vi "GetSourceOutput.vi"(7 "SMU":T1, 8 "Error In":errorcluster, 11 "Kiethley 2602 In":refnum<visa-resource-name>) -> (0 "Error Out":errorcluster, 2 "Enabled?":bool, 3 "Keithley 2602 Out":refnum<visa-resource-name>)   [LabVIEW 2012, in "Keithley-2602.lvlib"]
uses:
  Keithley-2602.lvlib
  Controls/SMU.ctl
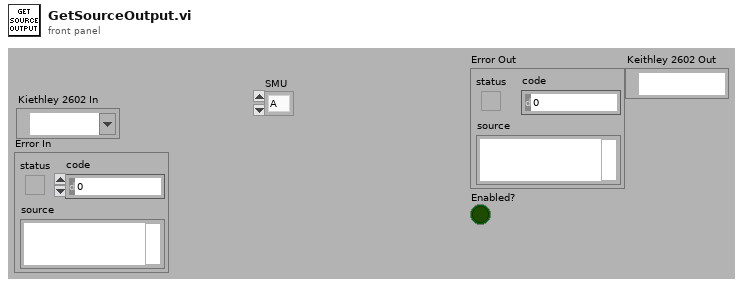
[diagram p1: front panel]
types:
  T1 = typedef "Keithley-2602.lvlib/SMU.ctl" = enum16{"A", "B"}
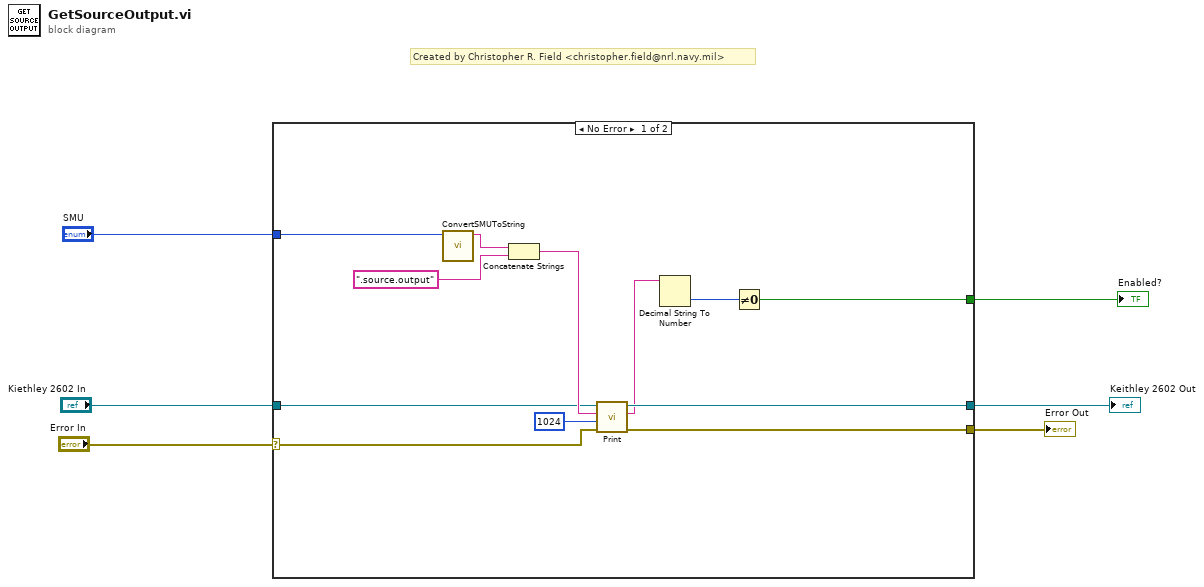
[diagram p0: block diagram]
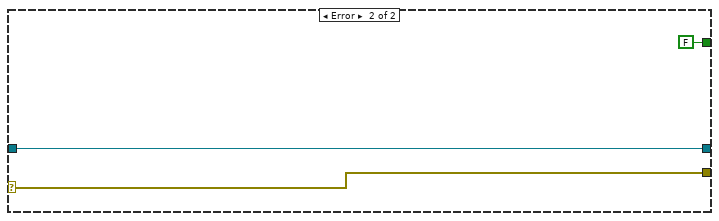
[diagram p2: hidden frame]
diagram:
  # "Created by Christopher R. Field <christopher.field@nrl.navy.mil>"
  n1 = case shown="No Error" "Error In" {
    selector: "Error In" -> [w7 w20]
    tunnel: "Kiethley 2602 In" -> [w14 w21]
    tunnel: [w13 w20] -> w5
    tunnel: [w12 w21] -> w4
    tunnel: [w9 FALSE] -> w3
    tunnel: "SMU" -> [w8 _]
    frame No Error {
      n2 = call "ConvertSMUToString.vi"("SMU"=w8) -> ("Channel"=w18:string)  [unwired: 10 in]
      n3 = Concatenate Strings(w18, ".source.output") -> (w16:string)
      n4 = call "Print.vi"("Error In"=w7, "Byte Count"=u32 1024, "Attribute"=w16, "Kiethley 2602 In"=w14) -> ("Error Out"=w13:errorcluster, "Output"=w11:string, "Keithley 2602 Out"=w12:refnum<visa-resource-name>)  [unwired: 5 in]
      n5 = Decimal String To Number(string=w11) -> (number=w10:i32)  [unwired: 2 in, 1 out]
      n6 = Not Equal To 0?(x=w10) -> (x != 0?=w9:bool)
    }
    frame Error {
    }
  }
  "Error Out" <- w5
  "Keithley 2602 Out" <- w4
  "Enabled?" <- w3
